vi "save_rx.vi"(3 "PA":dbl[][](array[numeric]), 4 "PB":dbl[][](array[numeric]), 5 "PC":dbl[][](array[numeric]), 6 "PATH":string, 8 "Tabsize":dbl, 10 "FreqTab":dbl[](array[numeric])) -> ()   [LabVIEW 2015]
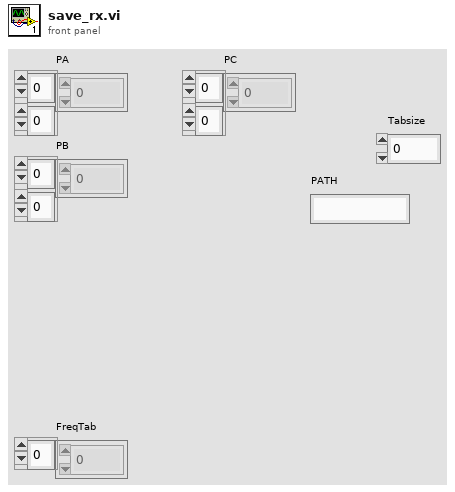
[diagram p1: front panel]
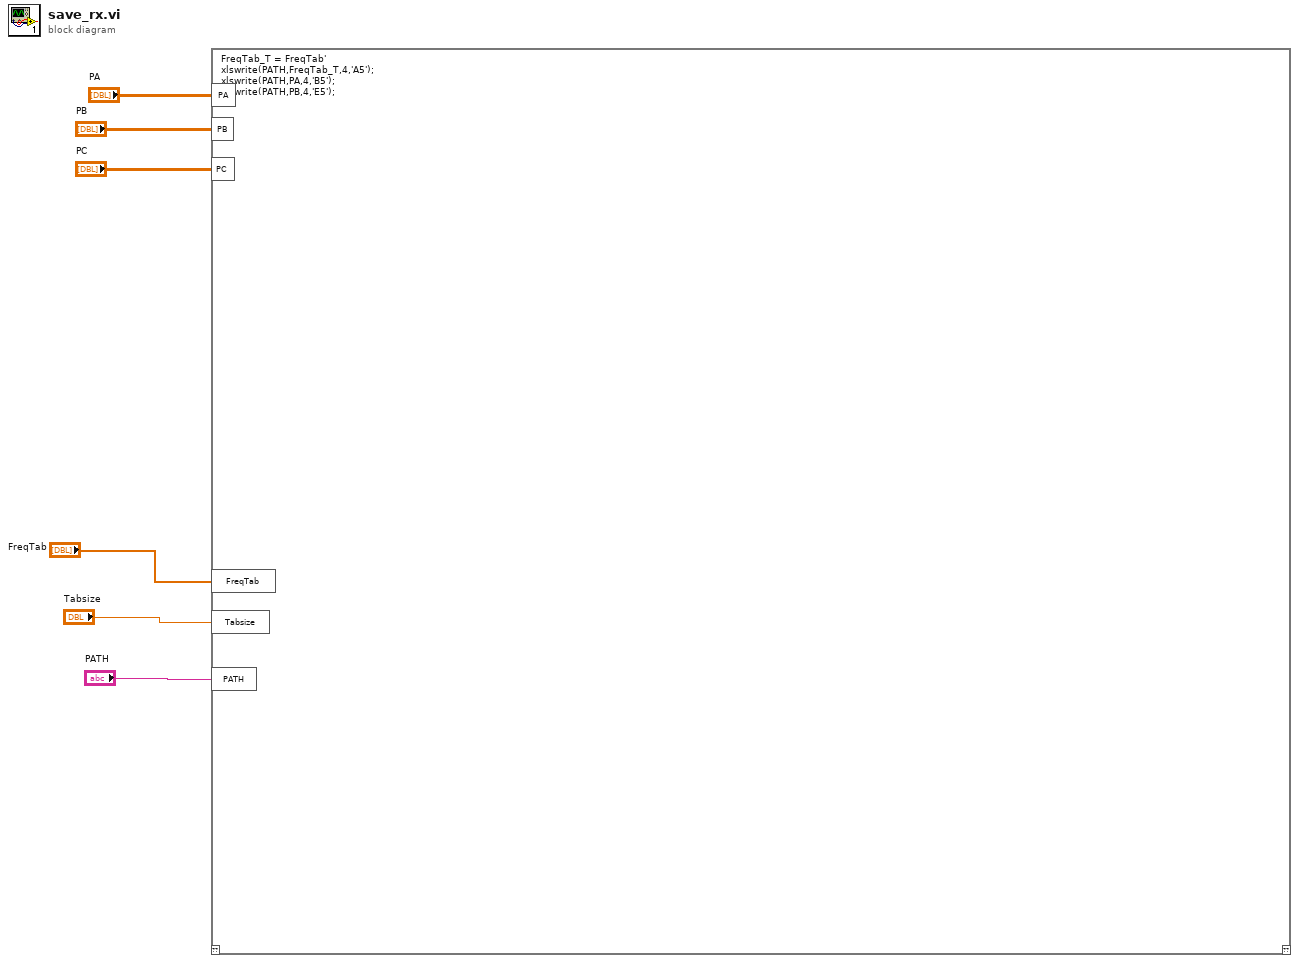
[diagram p0: block diagram]
diagram:
  n1 = script code="FreqTab_T = FreqTab'\nxlswrite(PATH,FreqTab_T,4,'A5');\nxlswrite(PATH,PA,4,'B5');\nxlswrite(PATH,PB,4,'E5');"("PA"="PA", "PB"="PB", "PC"="PC", "FreqTab"="FreqTab", "Tabsize"="Tabsize", "PATH"="PATH") -> ()  [unwired: 1 in, 1 out]
